vi "NIDCPower_channel_ganging - wait for event.vi"(8 "error in (no error)":errorcluster, 9 "event":T4=1030 items=["Source Complete Event"=1030, "Measure Complete Event"=1031, "Sequence Iteration Complete Event"=1032, "Sequence Engine Done Event"=1033, "Pulse Complete Event"=1051, "Ready For Pulse Trigger Event"=1052], 10 "timeout (10.0)":dbl=10.0, 11 "Ganged Session in":T1) -> (0 "error out":errorcluster, 3 "Ganged Session Out":T1)   [LabVIEW 2021]
uses:
  ctl/NIDCPower_channel_ganging - ctl - ganged config.ctl
  ctl/NIDCPower_channel_ganging - ctl - channel mode.ctl
  ctl/NIDCPower_channel_ganging - ctl - ganged session.ctl
  <instrlib>/niDCPower/nidcpower.llb/niDCPower Wait For Event - Event.ctl
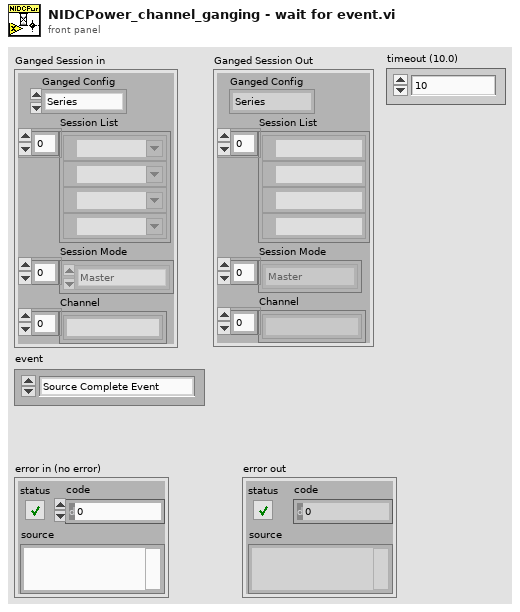
[diagram p1: front panel]
types:
  T1 = typedef "NIDCPower_channel_ganging - ctl - ganged session.ctl" = cluster{"Ganged Config":T2, "Session List":refnum<k15>[], "Session Mode":T3[], "Channel":string[]}
  T2 = typedef "NIDCPower_channel_ganging - ctl - ganged config.ctl" = enum16{"Series", "Parallel", "Manual"}
  T3 = typedef "NIDCPower_channel_ganging - ctl - channel mode.ctl" = enum16{"Master", "Slave", "Slave - Inverted"}
  T4 = typedef "niDCPower Wait For Event - Event.ctl" = i32
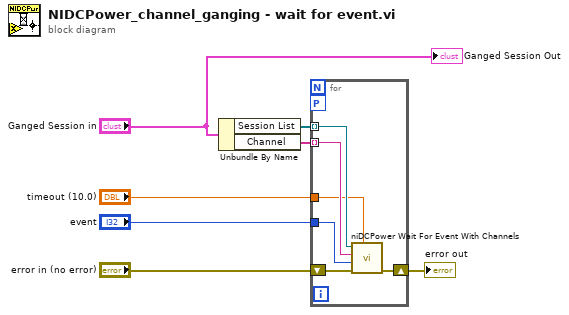
[diagram p0: block diagram]
diagram:
  n1 = Unbundle By Name("Ganged Session in") -> ("Session List"=w7:refnum<k15>[], "Channel"=w2:string[])
  n2 = for {
    tunnel: w7 -> [w11] mode=indexing
    shift-right: [w13] -> w6
    shift-left: "error in (no error)" -> [w12]
    workers-P: _ -> [_]
    tunnel: "event" -> [w10]
    tunnel: w2 -> [w9] mode=indexing
    tunnel: "timeout (10.0)" -> [w8]
    n3 = call <instrlib>:"niDCPower Wait For Event With Channels.vi"("timeout (10.0)"=w8, "error in (no error)"=w12, "event"=w10, "channel name"=w9, "instrument handle"=w11) -> ("error out"=w13:errorcluster)  [unwired: 5 in, 1 out]
  }
  "error out" <- w6
  "Ganged Session Out" <- "Ganged Session in"
